vi "EMAPRE_OFFLINE.vi"() -> ()   [LabVIEW 2015]
uses:
  <vilib>/Utility/file.llb/Read Delimited Spreadsheet (DBL).vi
panel:
  out "varience":dbl
  in  "?":bool
  out "Good Condition":bool
  out "Turn Fault":bool
  in  "RESULT":bool
  out "rms":dbl
  out "kurtosis":dbl
  out "Detail Coefficient 4":dbl[][](graph)
  in  "EXTRACT SIGNAL":bool
  in  "file path (dialog if empty)":path
  out "Signal Graph":dbl[][](graph)
  # "Stator Faults Detection on Induction Motor\n based on Electric Signals Measurement"
  # "Tiara Hardiyanti (3110151038)"
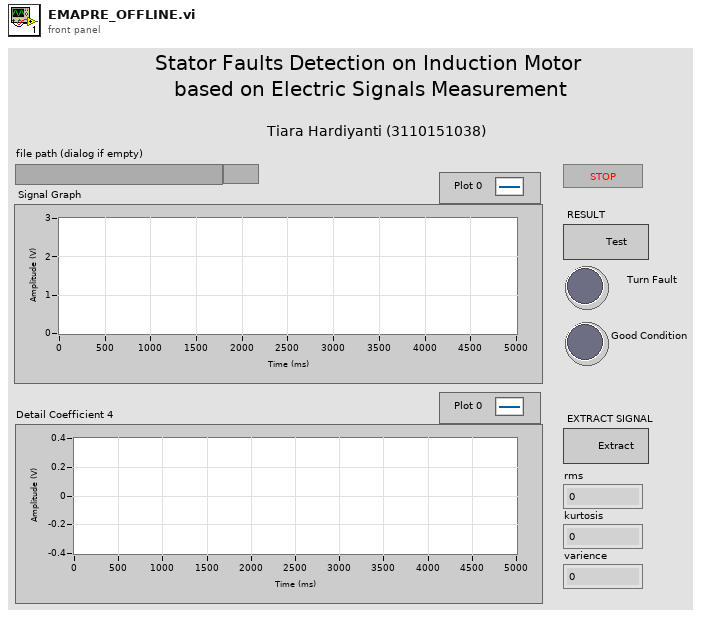
[diagram p1: front panel]
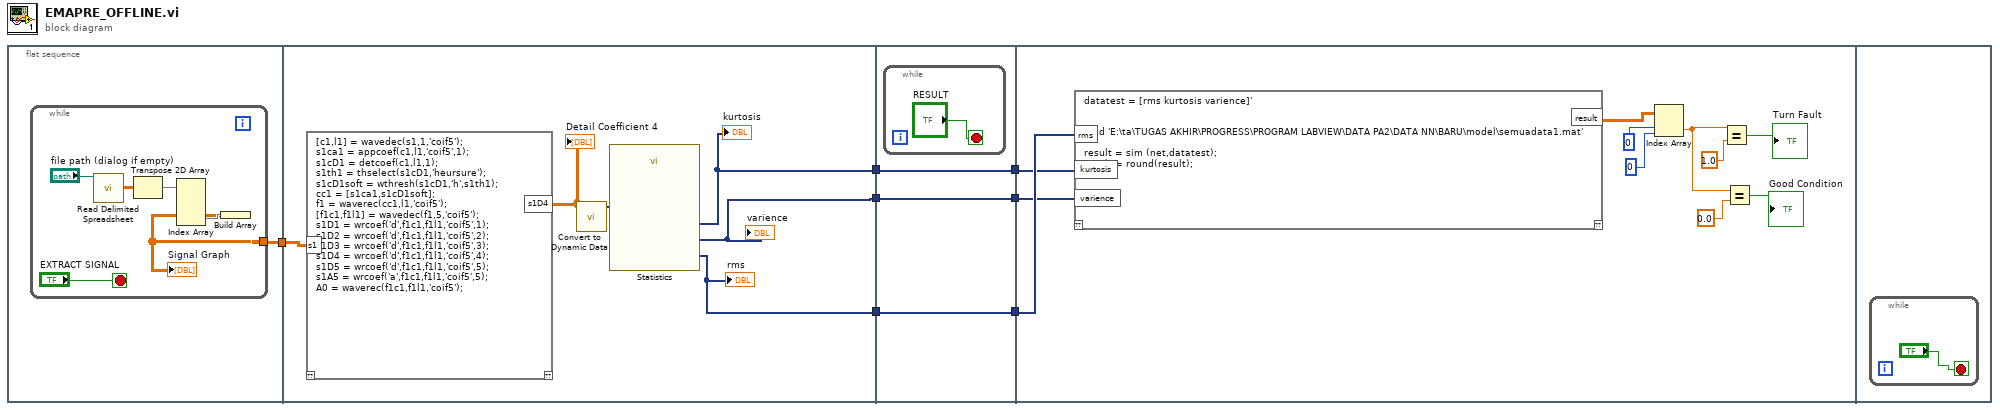
[diagram p0: block diagram]
diagram:
  n1 = flat-sequence {
    tunnel: [w8] -> w7
    tunnel: w7 -> [w20]
    tunnel: [w17] -> w6
    tunnel: [w16] -> w4
    tunnel: [w15] -> w2
    tunnel: w6 -> [w23]
    tunnel: [w23] -> w5
    tunnel: w4 -> [w22]
    tunnel: [w22] -> w3
    tunnel: w2 -> [w21]
    tunnel: [w21] -> w1
    tunnel: w5 -> [w27]
    tunnel: w3 -> [w26]
    tunnel: w1 -> [w25]
    frame #0 {
      n2 = while {
        tunnel: [w9] -> w8
        stop <- "EXTRACT SIGNAL" stop-if-true
        n3 = call-poly <vilib>:"Read Delimited Spreadsheet.vi"("file path (dialog if empty)"="file path (dialog if empty)") -> ("all rows"=w11:dbl[][])  [unwired: 9 in, 5 out]
        n4 = Transpose 2D Array(2D array=w11) -> (transposed array=w12:dbl[][])
        n5 = Index Array(array=w12) -> (element #2=w13:dbl[])  [unwired: 4 in, 1 out]
        n6 = Build Array(w13) -> (w9:dbl[][])
        "Signal Graph" <- w9
      }
    }
    frame #1 {
      n7 = script code="[c1,l1] = wavedec(s1,1,'coif5');\ns1ca1 = appcoef(c1,l1,'coif5',1);\ns1cD1 = detcoef(c1,l1,1);\ns1th1 = thselect(s1cD1,'heursure');\ns1cD1soft = wthresh(s1cD1,'h',s1th1);\ncc1 = [s1ca1,s1cD1soft];\nf1 = waverec(cc1,l1,'coif5');\n[f1c1,f1l1] = wavedec(f1,5,'coif5');\ns1D1 = wrcoef('d',f1c1,f1l1,'coif5',1);\ns1D2 = wrcoef('d',f1c1,f1l1,'coif5',2);\ns1D3 = wrcoef('d',f1c1,f1l1,'coif5',3);\ns1D4 = wrcoef('d',f1c1,f1l1,'coif5',4);\ns1D5 = wrcoef('d',f1c1,f1l1,'coif5',5);\ns1A5 = wrcoef('a',f1c1,f1l1,'coif5',5);\nA0 = waverec(f1c1,f1l1,'coif5');"("s1"=w20) -> ("s1D4"=w19:dbl[][])  [unwired: 1 in, 1 out]
      "Detail Coefficient 4" <- w19
      n8 = call "Convert to Dynamic Data"("2D Array"=w19) -> ("Dynamic Data Type"=w18:dynamicdata)  [unwired: 3 in]
      n9 = call "Statistics"("Signals"=w18) -> ("Kurtosis"=w16:dynamicdata, "Variance"=w15:dynamicdata, "RMS"=w17:dynamicdata)  [unwired: 23 in, 1 out]
      "kurtosis" <- w16
      "rms" <- w17
      "varience" <- w15
    }
    frame #2 {
      n10 = while {
        stop <- "RESULT" stop-if-true
      }
    }
    frame #3 {
      n11 = script code="datatest = [rms kurtosis varience]'\n\n\nload 'E:\\ta\\TUGAS AKHIR\\PROGRESS\\PROGRAM LABVIEW\\DATA PA2\\DATA NN\\BARU\\model\\semuadata1.mat'\n\nresult = sim (net,datatest);\nresult = round(result);"("kurtosis"=w26, "rms"=w27, "varience"=w25) -> ("result"=w31:dbl[][])  [unwired: 1 in, 1 out]
      n12 = Index Array(array=w31, index (row)=0 ("disabled index (row)"), index (col)=0 ("disabled index (col)")) -> (element=w28:dbl)
      n13 = Equal?(x=w28, y=1.0) -> (x = y?=→"Turn Fault":bool)
      n14 = Equal?(x=w28, y=0.0) -> (x = y?=→"Good Condition":bool)
    }
    frame #4 {
      n15 = while {
        stop <- "?" stop-if-true
      }
    }
  }
